vi "Reaction.vi"(5 "Enable potentiostat":bool, 6 "Experiment file path":path, 7 "Potentiostat channel":string(combo)="17158001", 8 "Enable rotation":bool, 9 "Rotation COM":refnum<visa-resource-name>="COM28", 10 "Control parameter":T1={"Pump 1 refill rate (ml/min) "=6.0, "Pump 1 refill volume (mL)"=1.8, "Pump 1 transfer rate (ml/min)"=0.08, "Pump 1 oscill. rate (ml/min)"=0.04, "Vertex potential 1(V)"=-0.5, "Initial potential (V)"=0.0, "Final potential (V)"=0.0, "Cycles"=1, "Delayed time for waiting(s)"=5.0, "Pressure (psi)"=15.0, "Vertex potential 2(V)"=0.0, "Use inital potential?"=TRUE, "Sample name"="", "To waste flow factor"=5.0, "Temperature (C)"=20.0, "Scan rate (V/s)"=10.0, "Use final potential?"=TRUE, "CV current range"="20MA", "Cell to use"="EXTERNAL"} {"Scan rate (V/s)" min=0.0 max=10.0 format="%#_4f"; "Vertex potential 2(V)" min=-5.0 max=5.0 format="%.3f"; "Cycles" min=1 max=30; "Final potential (V)" min=-5.0 format="%_3f"; "Initial potential (V)" min=-5.0 max=5.0 format="%.3f"; "Vertex potential 1(V)" min=-5.0 max=5.0 format="%.3f"; "Pump 1 oscill. rate (ml/min)" format="%#.4f"; "Pump 1 transfer rate (ml/min)" format="%#.4f"; "Pump 1 refill volume (mL)" format="%#.4f"; "Pump 1 refill rate (ml/min)" format="%#.4f"}, 11 "Configured COM ports":T2={"Pump 1 COM"="COM12", "Pump 2 COM"="COM9", "Pump 3 COM"="COM13", "Pump 4 COM"="COM4", "Pump 5 COM"="COM15"}) -> ()   [LabVIEW 2017]
uses:
  C:/Program Files (x86)/Princeton Applied Research/VersaSTAT Development Kit/LabView v2011 Examples/VersaSTATControl.dll
  Program Files (x86)/Princeton Applied Research/VersaSTAT Development Kit/LabView v2011 Examples/VersaSTATControl.dll
  <instrlib>/Harvard Apparatus PHD Ultra Series/Harvard Apparatus PHD Ultra Series.lvlib
  <instrlib>/Princeton potentiostat/Princeton potentiostat.lvlib
panel:
  out "Cell to use":string
  out "CV current range":string
  out "Scan rate (V/s)":dbl
  out "Cycles":i32
  out "Vertex potential 1(V)":dbl
  out "Vertex potential 2(V)":dbl
  out "Initial potential (V)":dbl
  out "Use final potential?":bool
  out "Potentiostat ref.":refnum<k24>
  out "Connect":bool
  out "Temperature (C)":dbl
  out "To waste flow factor":dbl
  out "Sample name":string
  out "Use initial potential?":bool
  out "Pump 5 COM":refnum<visa-resource-name>="COM12"
  out "Final voltage (V)":dbl min=-6.0 max=6.0 format="%.3f"
  out "Pressure (psi)":dbl=15.0
  out "Delayed time for waiting(s)":dbl
  out "Pump 4 COM":refnum<visa-resource-name>="COM12"
  out "Pump 3 COM":refnum<visa-resource-name>="COM12"
  out "Pump 2 COM":refnum<visa-resource-name>="COM12"
  out "Pump 1 COM":refnum<visa-resource-name>="COM12"
  out "Pump 1 oscill. rate (ml/min)":dbl=0.5 format="%#.4f"
  out "Pump 1 transfer rate (ml/min)":dbl=0.15 format="%#.4f"
  out "Pump 1 refill volume (mL)":dbl=1.0 format="%#.4f"
  out "Pump 1 refill rate (ml/min)":dbl=6.0 format="%#.4f"
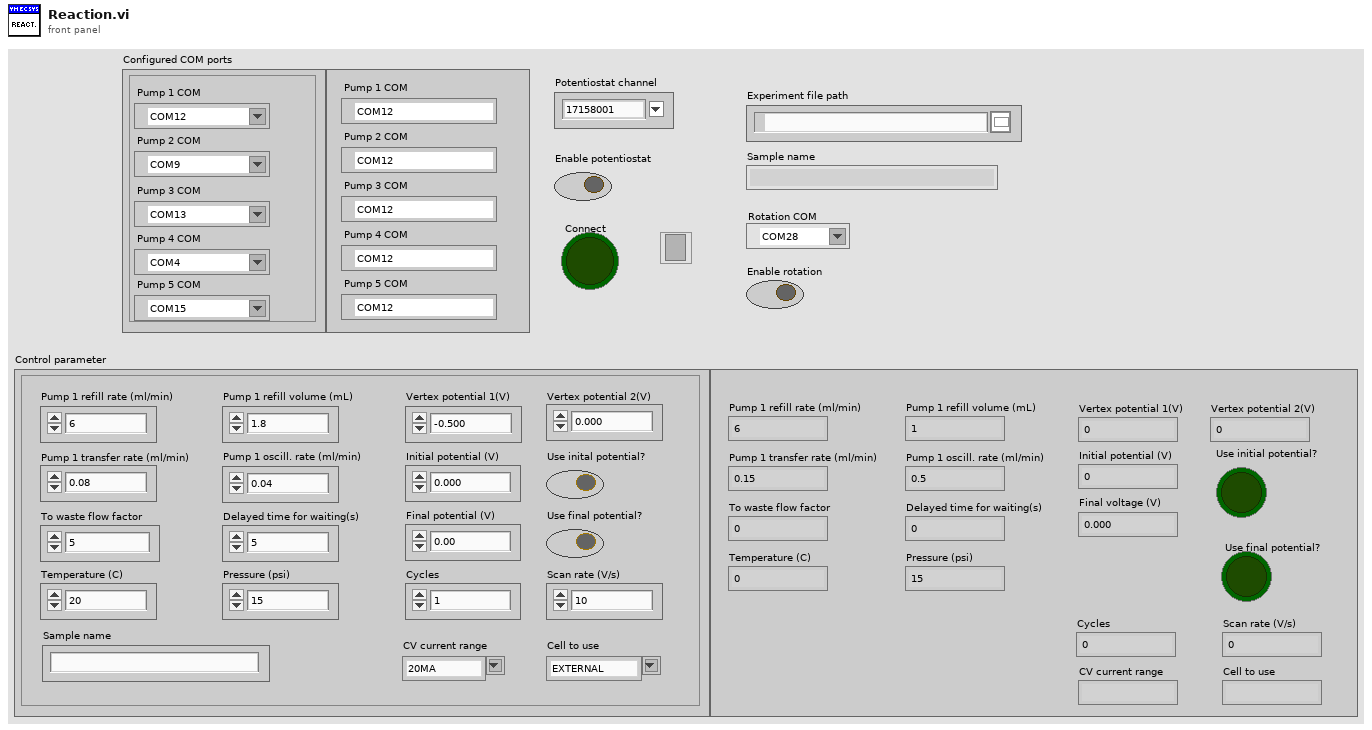
[diagram p1: front panel]
types:
  T1 = cluster{"Pump 1 refill rate (ml/min) ":dbl, "Pump 1 refill volume (mL)":dbl, "Pump 1 transfer rate (ml/min)":dbl, "Pump 1 oscill. rate (ml/min)":dbl, "Vertex potential 1(V)":dbl, "Initial potential (V)":dbl, "Final potential (V)":dbl, "Cycles":i32, "Delayed time for waiting(s)":dbl, "Pressure (psi)":dbl, "Vertex potential 2(V)":dbl, "Use inital potential?":bool, "Sample name":string, "To waste flow factor":dbl, "Temperature (C)":dbl, "Scan rate (V/s)":dbl, "Use final potential?":bool, "CV current range":string, "Cell to use":string}
  T2 = cluster{"Pump 1 COM":refnum<visa-resource-name>, "Pump 2 COM":refnum<visa-resource-name>, "Pump 3 COM":refnum<visa-resource-name>, "Pump 4 COM":refnum<visa-resource-name>, "Pump 5 COM":refnum<visa-resource-name>}
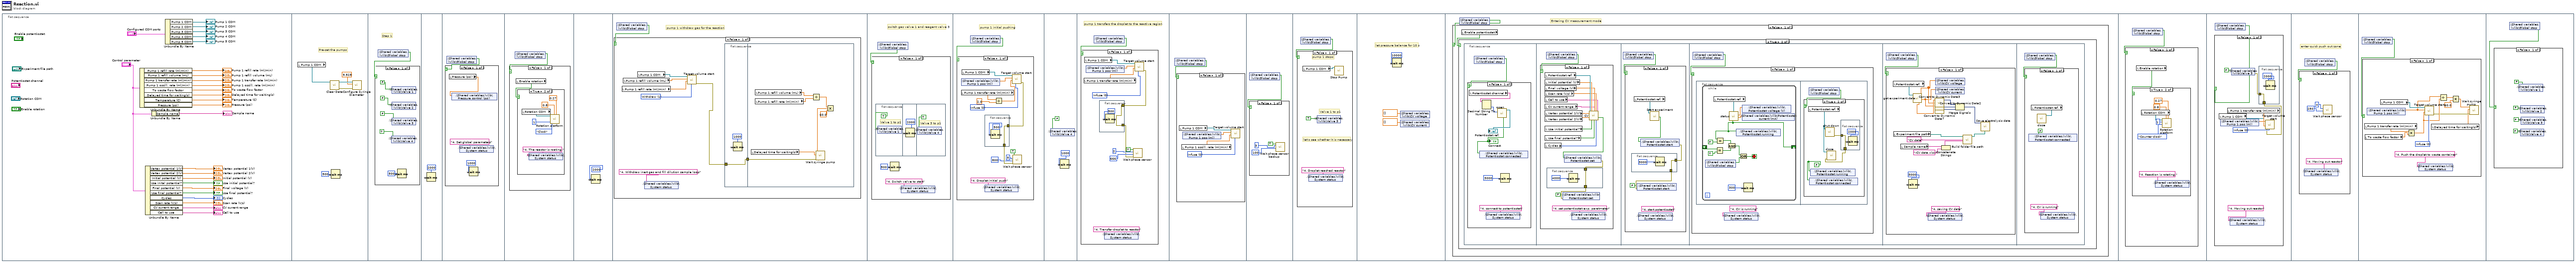
[diagram p0: block diagram]
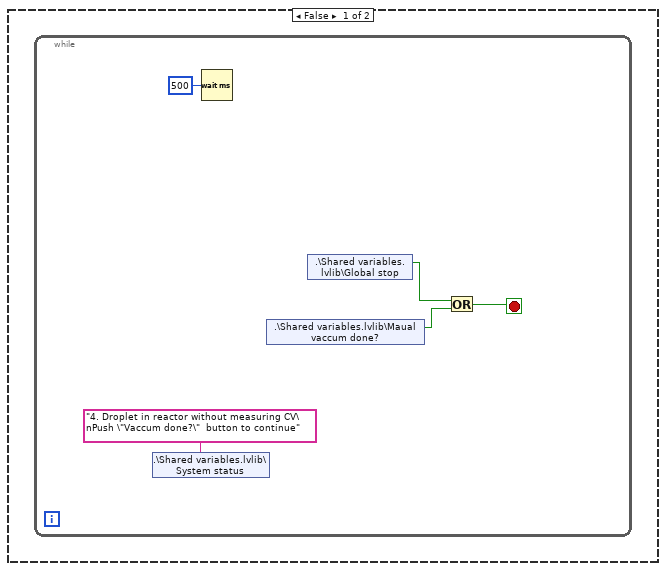
[diagram p13: hidden frame]
diagram:
  n1 = flat-sequence {
    frame #0 {
      n2 = Unbundle By Name("Control parameter") -> ("Pump 1 refill rate (ml/min)"=→"Pump 1 refill rate (ml/min)":dbl, "Pump 1 refill volume (mL)"=→"Pump 1 refill volume (mL)":dbl, "Pump 1 transfer rate (ml/min)"=→"Pump 1 transfer rate (ml/min)":dbl, "Pump 1 oscill. rate (ml/min)"=→"Pump 1 oscill. rate (ml/min)":dbl, "To waste flow factor"=→"To waste flow factor":dbl, "Delayed time for waiting(s)"=→"Delayed time for waiting(s)":dbl, "Temperature (C)"=→"Temperature (C)":dbl, "Pressure (psi)"=→"Pressure (psi)":dbl)
      n3 = Unbundle By Name("Control parameter") -> ("Vertex potential 1(V)"=→"Vertex potential 1(V)":dbl, "Vertex potential 2(V)"=→"Vertex potential 2(V)":dbl, "Initial potential (V)"=→"Initial potential (V)":dbl, "Use inital potential?"=→"Use initial potential?":bool, "Final potential (V)"=→"Final voltage (V)":dbl, "Use final potential?"=→"Use final potential?":bool, "Cycles"=→"Cycles":i32, "Scan rate (V/s)"=→"Scan rate (V/s)":dbl, "CV current range"=→"CV current range":string, "Cell to use"=→"Cell to use":string)
      n4 = Unbundle By Name("Control parameter") -> ("Sample name"=→"Sample name":string)
      n5 = Unbundle By Name("Configured COM ports") -> ("Pump 1 COM"=→"Pump 1 COM":refnum<visa-resource-name>, "Pump 2 COM"=→"Pump 2 COM":refnum<visa-resource-name>, "Pump 3 COM"=→"Pump 3 COM":refnum<visa-resource-name>, "Pump 4 COM"=→"Pump 4 COM":refnum<visa-resource-name>, "Pump 5 COM"=→"Pump 5 COM":refnum<visa-resource-name>)
    }
    frame #1 {
      # "Pre-set the pumps"
      n6 = local read "Pump 1 COM"() -> (w31:refnum<visa-resource-name>)
      n7 = call <instrlib>:"Clear Data.vi"("VISA resource name"=w31) -> ("error out"=w29:errorcluster, "VISA resource name out"=w30:refnum<visa-resource-name>)  [unwired: 9 in]
      n8 = Wait (ms)(milliseconds to wait=u32 500) -> ()  [unwired: 1 out]
      n9 = call <instrlib>:"Configure Syringe Diameter.vi"("error in (no error)"=w29, "Syringe Diameter (20 mm)"=9.525, "VISA resource name"=w30) -> ()  [unwired: 7 in, 2 out]
    }
    frame #2 {
      # "Step 1"
      n10 = shared-variable ".\\Shared variables.lvlib\\Global stop"() -> (w32:bool)  [unwired: 1 in, 1 out]
      n11 = case shown="False" w32 {
        frame False {
          n12 = shared-variable ".\\Shared variables.lvlib\\Valve 4"(TRUE) -> ()  [unwired: 1 in, 1 out]
          n13 = shared-variable ".\\Shared variables.lvlib\\Valve 1"(FALSE) -> ()  [unwired: 1 in, 1 out]
          n14 = shared-variable ".\\Shared variables.lvlib\\Valve 2"(FALSE) -> ()  [unwired: 1 in, 1 out]
          n15 = shared-variable ".\\Shared variables.lvlib\\Valve 3"(FALSE) -> ()  [unwired: 1 in, 1 out]
          n16 = Wait (ms)(milliseconds to wait=u32 500) -> ()  [unwired: 1 out]
        }
        frame True {
        }
      }
    }
    frame #3 {
      n17 = Wait (ms)(milliseconds to wait=u32 2000) -> ()  [unwired: 1 out]
    }
    frame #4 {
      n18 = shared-variable ".\\Shared variables.lvlib\\Global stop"() -> (w39:bool)  [unwired: 1 in, 1 out]
      n19 = case shown="False" w39 {
        frame False {
          n20 = local read "Pressure (psi)"() -> (w42:dbl)
          n21 = shared-variable ".\\Shared variables.lvlib\\Pressure control (psi)"(w42) -> ()  [unwired: 1 in, 1 out]
          n22 = shared-variable ".\\Shared variables.lvlib\\System status"("4. Set global parameters" ("System status")) -> ()  [unwired: 1 in, 1 out]
          n23 = Wait (ms)(milliseconds to wait=u32 1000) -> ()  [unwired: 1 out]
        }
        frame True {
        }
      }
    }
    frame #5 {
      n24 = shared-variable ".\\Shared variables.lvlib\\Global stop"() -> (w43:bool)  [unwired: 1 in, 1 out]
      n25 = case shown="False" w43 {
        frame False {
          n26 = local read "Enable rotation"() -> (w44:bool)
          n27 = case shown="True" w44 {
            frame False {
            }
            frame True {
              n28 = local read "Rotation COM"() -> (w46:refnum<visa-resource-name>)
              n29 = shared-variable ".\\Shared variables.lvlib\\System status"("4. The reactor is roating." ("System status")) -> ()  [unwired: 1 in, 1 out]
              n30 = call "Rotation platform.vi"("Revolution (0-0.5)"=0.27, "Rotation speed (RPM)"=0.8, "Direction"=enum16{"Counter clock", "Clock"}."Clock", "Pump number"=1, "Rotation COM"=w46) -> ()  [unwired: 7 in]
            }
          }
        }
        frame True {
        }
      }
    }
    frame #6 {
      n31 = Wait (ms)(milliseconds to wait=u32 2000) -> ()  [unwired: 1 out]
    }
    frame #7 {
      # "pump 1 withdraw gas for the reaction"
      n32 = shared-variable ".\\Shared variables.lvlib\\Global stop"() -> (w52:bool)  [unwired: 1 in, 1 out]
      n33 = case shown="False" w52 {
        frame False {
          w56 = u16 1 items=["Infuse", "Withdraw"] ("Pump Direction (0:Infuse)")
          n34 = local read "Pump 1 refill rate (ml/min)"() -> (w57:dbl)
          n35 = local read "Pump 1 refill volume (mL)"() -> (w58:dbl)
          n36 = local read "Pump 1 COM"() -> (w55:refnum<visa-resource-name>)
          n37 = shared-variable ".\\Shared variables.lvlib\\System status"("4. Withdraw inert gas and fill dilution sample loop" ("System status")) -> ()  [unwired: 1 in, 1 out]
          n38 = call "Target volume start.vi"("Pump Direction (0:Infuse)"=w56, "Flow Rate (ml/min)"=w57, "Target volume (ml)"=w58, "VISA resource name"=w55) -> ("error out"=w53:errorcluster)  [unwired: 6 in, 1 out]
          n39 = flat-sequence {
            tunnel: [w60] -> w59
            tunnel: w53 -> [w60]
            tunnel: w59 -> [w66]
            frame #0 {
              n40 = Wait (ms)(milliseconds to wait=u32 1000) -> ()  [unwired: 1 out]
            }
            frame #1 {
              n41 = local read "Delayed time for waiting(s)"() -> (w65:dbl)
              n42 = local read "Pump 1 refill volume (mL)"() -> (w68:dbl)
              n43 = local read "Pump 1 refill rate (ml/min)"() -> (w67:dbl)
              n44 = Divide(x=w68, y=w67) -> (x/y=w62:dbl)
              n45 = Multiply(x=w62, y=60.0) -> (x*y=w64:dbl)
              n46 = call "Wait syringe pump.vi"("error in (no error)"=w66, "Delayed time (s)"=w65, "Time Target (s)"=w64) -> ()  [unwired: 8 in, 1 out]
            }
          }
        }
        frame True {
        }
      }
    }
    frame #8 {
      # "switch gas valve 1 and reagent valve 3"
      n47 = shared-variable ".\\Shared variables.lvlib\\Global stop"() -> (w69:bool)  [unwired: 1 in, 1 out]
      n48 = case shown="False" w69 {
        frame False {
          n49 = flat-sequence {
            frame #0 {
              # "Valve 1 to p1"
              n50 = shared-variable ".\\Shared variables.lvlib\\Valve 1"(TRUE) -> ()  [unwired: 1 in, 1 out]
            }
            frame #1 {
              n51 = Wait (ms)(milliseconds to wait=u32 2000) -> ()  [unwired: 1 out]
            }
            frame #2 {
              # "Valve 3 to p1"
              n52 = shared-variable ".\\Shared variables.lvlib\\Valve 4"(TRUE) -> ()  [unwired: 1 in, 1 out]
            }
          }
          n53 = Wait (ms)(milliseconds to wait=u32 500) -> ()  [unwired: 1 out]
          n54 = shared-variable ".\\Shared variables.lvlib\\System status"("4. Switch valve to start" ("System status")) -> ()  [unwired: 1 in, 1 out]
        }
        frame True {
        }
      }
    }
    frame #9 {
      # "pump 1 initial pushing"
      n55 = shared-variable ".\\Shared variables.lvlib\\Global stop"() -> (w75:bool)  [unwired: 1 in, 1 out]
      n56 = case shown="False" w75 {
        frame False {
          w87 = u16 0 items=["Infuse", "Withdraw"] ("Pump Direction (0:Infuse)")
          n57 = shared-variable ".\\Shared variables.lvlib\\Pump 1 pos (ml)"() -> (w78:dbl)  [unwired: 1 in, 1 out]
          n58 = local read "Pump 1 transfer rate (ml/min)"() -> (w83:dbl)
          n59 = local read "Pump 1 COM"() -> (w86:refnum<visa-resource-name>)
          n60 = flat-sequence {
            tunnel: [w88] -> w82
            tunnel: w81 -> [w88]
            frame #0 {
              n61 = Wait (ms)(milliseconds to wait=u32 500) -> ()  [unwired: 1 out]
            }
          }
          n62 = shared-variable ".\\Shared variables.lvlib\\System status"("4. Droplet initial push" ("System status")) -> ()  [unwired: 1 in, 1 out]
          n63 = Divide(x=w83, y=2.0) -> (x/y=w85:dbl)
          n64 = call "Target volume start.vi"("Pump Direction (0:Infuse)"=w87, "Flow Rate (ml/min)"=w85, "Target volume (ml)"=w78, "VISA resource name"=w86) -> ("error out"=w81:errorcluster)  [unwired: 6 in, 1 out]
          n65 = call "Wait phase sensor.vi"("error in (no error)"=w82, "Sensitivity time (ms)"=u32 800 ("milliseconds to wait"), "Phase sensor number"=5, "Sense T/F"=TRUE) -> ()  [unwired: 7 in, 1 out]
        }
        frame True {
        }
      }
    }
    frame #10 {
      n66 = shared-variable ".\\Shared variables.lvlib\\Valve 4"(FALSE) -> ()  [unwired: 1 in, 1 out]
      n67 = Wait (ms)(milliseconds to wait=u32 1000) -> ()  [unwired: 1 out]
    }
    frame #11 {
      # "pump 1 transfers the droplet to the reactive region"
      n68 = shared-variable ".\\Shared variables.lvlib\\Global stop"() -> (w92:bool)  [unwired: 1 in, 1 out]
      n69 = case shown="False" w92 {
        frame False {
          w102 = u16 0 items=["Infuse", "Withdraw"] ("Pump Direction (0:Infuse)")
          n70 = local read "Pump 1 transfer rate (ml/min)"() -> (w100:dbl)
          n71 = local read "Pump 1 COM"() -> (w101:refnum<visa-resource-name>)
          n72 = shared-variable ".\\Shared variables.lvlib\\Pump 1 pos (ml)"() -> (w99:dbl)  [unwired: 1 in, 1 out]
          n73 = flat-sequence {
            tunnel: [w103] -> w93
            tunnel: w98 -> [w103]
            frame #0 {
              n74 = Wait (ms)(milliseconds to wait=u32 500) -> ()  [unwired: 1 out]
            }
          }
          n75 = shared-variable ".\\Shared variables.lvlib\\System status"("4. Transfer droplet to reactor" ("System status")) -> ()  [unwired: 1 in, 1 out]
          n76 = call "Wait phase sensor.vi"("error in (no error)"=w93, "Sensitivity time (ms)"=u32 666 ("milliseconds to wait"), "Phase sensor number"=2, "Sense T/F"=TRUE) -> ()  [unwired: 7 in, 1 out]
          n77 = call "Target volume start.vi"("Pump Direction (0:Infuse)"=w102, "Flow Rate (ml/min)"=w100, "Target volume (ml)"=w99, "VISA resource name"=w101) -> ("error out"=w98:errorcluster)  [unwired: 6 in, 1 out]
        }
        frame True {
        }
      }
    }
    frame #12 {
      n78 = shared-variable ".\\Shared variables.lvlib\\Global stop"() -> (w105:bool)  [unwired: 1 in, 1 out]
      n79 = case shown="False" w105 {
        frame False {
          w106 = u16 0 items=["Infuse", "Withdraw"] ("Pump Direction (0:Infuse)")
          n80 = local read "Pump 1 COM"() -> (w109:refnum<visa-resource-name>)
          n81 = local read "Pump 1 oscill. rate (ml/min)"() -> (w108:dbl)
          n82 = shared-variable ".\\Shared variables.lvlib\\Pump 1 pos (ml)"() -> (w107:dbl)  [unwired: 1 in, 1 out]
          n83 = call "Target volume start.vi"("Pump Direction (0:Infuse)"=w106, "Flow Rate (ml/min)"=w108, "Target volume (ml)"=w107, "VISA resource name"=w109) -> ()  [unwired: 6 in, 2 out]
        }
        frame True {
        }
      }
    }
    frame #13 {
      n84 = shared-variable ".\\Shared variables.lvlib\\Global stop"() -> (w110:bool)  [unwired: 1 in, 1 out]
      n85 = case shown="False" w110 {
        frame False {
          n86 = call "Wait phase sensor backup.vi"("Sensitivity time (ms)"=u32 100 ("milliseconds to wait"), "Phase sensor number"=3, "Sense T/F"=TRUE) -> ()  [unwired: 8 in, 1 out]
        }
        frame True {
        }
      }
    }
    frame #14 {
      n87 = shared-variable ".\\Shared variables.lvlib\\Global stop"() -> (w114:bool)  [unwired: 1 in, 1 out]
      n88 = case shown="False" w114 {
        frame False {
          # "Valve 1 to p1"
          # "let's see whether it is necessary"
          # "pump 1 stops"
          n89 = local read "Pump 1 COM"() -> (w116:refnum<visa-resource-name>)
          n90 = shared-variable ".\\Shared variables.lvlib\\System status"("4. Droplet reached reactor" ("System status")) -> ()  [unwired: 1 in, 1 out]
          n91 = shared-variable ".\\Shared variables.lvlib\\Valve 3"(TRUE) -> ()  [unwired: 1 in, 1 out]
          n92 = call <instrlib>:"Stop Pump.vi"("VISA resource name"=w116) -> ()  [unwired: 9 in, 2 out]
        }
        frame True {
        }
      }
    }
    frame #15 {
      # "let pressure balance for 10 s"
      n93 = Wait (ms)(milliseconds to wait=u32 10000) -> ()  [unwired: 1 out]
      n94 = shared-variable ".\\Shared variables.lvlib\\CV voltage"(dbl[] [] ("CV voltage")) -> ()  [unwired: 1 in, 1 out]
      n95 = shared-variable ".\\Shared variables.lvlib\\CV current"(dbl[] [] ("CV current")) -> ()  [unwired: 1 in, 1 out]
    }
    frame #16 {
      # "Entering CV measurement mode"
      n96 = shared-variable ".\\Shared variables.lvlib\\Global stop"() -> (w121:bool)  [unwired: 1 in, 1 out]
      n97 = case shown="False" w121 {
        frame False {
          n98 = local read "Enable potentiostat"() -> (w122:bool)
          n99 = case shown="True" w122 {
            frame False {
              n100 = while {
                stop <- w123 stop-if-true
                n101 = shared-variable ".\\Shared variables.lvlib\\System status"("4. Droplet in reactor without measuring CV\nPush \"Vaccum done?\"  button to continue" ("System status")) -> ()  [unwired: 1 in, 1 out]
                n102 = Wait (ms)(milliseconds to wait=u32 500) -> ()  [unwired: 1 out]
                n103 = shared-variable ".\\Shared variables.lvlib\\Maual vaccum done?"() -> (w124:bool)  [unwired: 1 in, 1 out]
                n104 = shared-variable ".\\Shared variables.lvlib\\Global stop"() -> (w125:bool)  [unwired: 1 in, 1 out]
                n105 = Or(x=w125, y=w124) -> (x .or. y?=w123:bool)
              }
            }
            frame True {
              n106 = flat-sequence {
                frame #0 {
                  n107 = shared-variable ".\\Shared variables.lvlib\\Global stop"() -> (w128:bool)  [unwired: 1 in, 1 out]
                  n108 = case shown="False" w128 {
                    frame False {
                      n109 = local read "Potentiostat channel"() -> (w131:string)
                      n110 = Decimal String To Number(string=w131) -> (number=w134:i32)  [unwired: 2 in, 1 out]
                      n111 = shared-variable ".\\Shared variables.lvlib\\System status"("4. connect to potentiostat" ("System status")) -> ()  [unwired: 1 in, 1 out]
                      n112 = call <instrlib>:"open.vi"("iSerialNumber"=w134) -> ("Connect"=w132:bool, "reference out"=→"Potentiostat ref.":refnum<k24>)  [unwired: 7 in, 2 out]
                      "Connect" <- w132
                      n113 = shared-variable ".\\Shared variables.lvlib\\Potentiostat connected"(w132) -> ()  [unwired: 1 in, 1 out]
                      n114 = Wait (ms)(milliseconds to wait=u32 3000) -> ()  [unwired: 1 out]
                    }
                    frame True {
                    }
                  }
                }
                frame #1 {
                  n115 = shared-variable ".\\Shared variables.lvlib\\Global stop"() -> (w135:bool)  [unwired: 1 in, 1 out]
                  n116 = case shown="False" w135 {
                    frame False {
                      n117 = local read "Potentiostat ref."() -> (w151:refnum<k24>)
                      n118 = local read "Initial potential (V)"() -> (w148:dbl)
                      n119 = local read "Final voltage (V)"() -> (w147:dbl)
                      n120 = local read "Scan rate (V/s)"() -> (w146:dbl)
                      n121 = local read "Cell to use"() -> (w145:string)
                      n122 = local read "CV current range"() -> (w144:string)
                      n123 = local read "Vertex potential 1(V)"() -> (w143:dbl)
                      n124 = local read "Vertex potential 2(V)"() -> (w142:dbl)
                      n125 = local read "Use initial potential?"() -> (w141:bool)
                      n126 = local read "Use final potential?"() -> (w140:bool)
                      n127 = local read "Cycles"() -> (w139:i32)
                      n128 = flat-sequence {
                        tunnel: [w152] -> w138
                        tunnel: w137 -> [w152]
                        frame #0 {
                          n129 = Wait (ms)(milliseconds to wait=u32 4000) -> ()  [unwired: 1 out]
                        }
                      }
                      n130 = shared-variable ".\\Shared variables.lvlib\\Potentiostat set"(FALSE ("Potentiostat set"), error in=w138) -> ()  [unwired: 1 out]
                      n131 = shared-variable ".\\Shared variables.lvlib\\System status"("4. set potentiostat exp. paratmeter" ("System status")) -> ()  [unwired: 1 in, 1 out]
                      n132 = call <instrlib>:"CV.vi"("reference"=w151, "Vertex potential 1 (V)"=w143, "Vertex potential 2 (V)"=w142, "Initial potential (V)"=w148, "Use initial potential?"=w141, "Final potential (V)"=w147, "Use final potential?"=w140, "Scan rate (V/s)"=w146, "Cycles"=w139, "Cell to use"=w145, "Current range"=w144) -> ("Experiment setup correctly"=w150:bool)  [unwired: 5 in, 3 out]
                      n133 = shared-variable ".\\Shared variables.lvlib\\Potentiostat set"(w150) -> (error out=w137:errorcluster)  [unwired: 1 in]
                    }
                    frame True {
                    }
                  }
                }
                frame #2 {
                  n134 = shared-variable ".\\Shared variables.lvlib\\Global stop"() -> (w154:bool)  [unwired: 1 in, 1 out]
                  n135 = case shown="False" w154 {
                    frame False {
                      n136 = flat-sequence {
                        tunnel: [w161] -> w157
                        tunnel: w156 -> [w161]
                        frame #0 {
                          n137 = Wait (ms)(milliseconds to wait=u32 3000) -> ()  [unwired: 1 out]
                        }
                      }
                      n138 = local read "Potentiostat ref."() -> (w160:refnum<k24>)
                      n139 = shared-variable ".\\Shared variables.lvlib\\Potentiostat start"(FALSE ("Potentiostat start"), error in=w157) -> ()  [unwired: 1 out]
                      n140 = shared-variable ".\\Shared variables.lvlib\\System status"("4. start potentiostat" ("System status")) -> ()  [unwired: 1 in, 1 out]
                      n141 = call <instrlib>:"Start experiment.vi"("reference"=w160) -> ("Start"=w159:bool)  [unwired: 9 in, 1 out]
                      n142 = shared-variable ".\\Shared variables.lvlib\\Potentiostat start"(w159) -> (error out=w156:errorcluster)  [unwired: 1 in]
                    }
                    frame True {
                    }
                  }
                }
                frame #3 {
                  n143 = shared-variable ".\\Shared variables.lvlib\\Global stop"() -> (w163:bool)  [unwired: 1 in, 1 out]
                  n144 = case shown="False" w163 {
                    frame False {
                      n145 = flat-sequence {
                        frame #0 {
                          n146 = while {
                            shift-right: [w176] -> _
                            shift-left: _ -> [w174]
                            stop <- w168 stop-if-true
                            n147 = shared-variable ".\\Shared variables.lvlib\\Global stop"() -> (w169:bool)  [unwired: 1 in, 1 out]
                            n148 = local read "Potentiostat ref."() -> (w177:refnum<k24>)
                            n149 = Equal?(x=w174, y=TRUE) -> (x = y?=w171:bool)
                            n150 = call <instrlib>:"status.vi"("reference"=w177) -> ("Current (A)"=w166:dbl, "Voltage (V)"=w167:dbl, "Experiment running"=w176:bool)  [unwired: 4 in, 4 out]
                            n151 = Equal?(x=w176, y=FALSE) -> (x = y?=w172:bool)
                            n152 = And(x=w172, y=w171) -> (x .and. y?=w170:bool)
                            n153 = shared-variable ".\\Shared variables.lvlib\\Potentiostat running"(w176) -> ()  [unwired: 1 in, 1 out]
                            n154 = Or(x=w170, y=w169) -> (x .or. y?=w168:bool)
                            n155 = shared-variable ".\\Shared variables.lvlib\\Potentiostat voltage (V)"(w167) -> ()  [unwired: 1 in, 1 out]
                            n156 = shared-variable ".\\Shared variables.lvlib\\Potentiostat current (mA)"(w166) -> ()  [unwired: 1 in, 1 out]
                            n157 = Wait (ms)(milliseconds to wait=u32 300) -> ()  [unwired: 1 out]
                          }
                        }
                        frame #1 {
                          n158 = shared-variable ".\\Shared variables.lvlib\\Global stop"() -> (w178:bool)  [unwired: 1 in, 1 out]
                          n159 = case shown="True" w178 {
                            frame False {
                            }
                            frame True {
                              w182 = FALSE ("Potentiostat running")
                              n160 = local read "Potentiostat ref."() -> (w181:refnum<k24>)
                              n161 = shared-variable ".\\Shared variables.lvlib\\Potentiostat connected"(w182) -> ()  [unwired: 1 in, 1 out]
                              n162 = shared-variable ".\\Shared variables.lvlib\\Potentiostat running"(w182) -> ()  [unwired: 1 in, 1 out]
                              n163 = call <instrlib>:"shut down.vi"("reference"=w181) -> ("error out"=w179:errorcluster)  [unwired: 10 in]
                              n164 = call <instrlib>:"close.vi"("error in (no error)"=w180, "reference"=w181) -> ()  [unwired: 9 in, 1 out]
                              n165 = flat-sequence {
                                tunnel: [w183] -> w180
                                tunnel: w179 -> [w183]
                                frame #0 {
                                n166 = Wait (ms)(milliseconds to wait=u32 2000) -> ()  [unwired: 1 out]
                                }
                              }
                            }
                          }
                        }
                      }
                      n167 = shared-variable ".\\Shared variables.lvlib\\System status"("4. CV is running" ("System status")) -> ()  [unwired: 1 in, 1 out]
                    }
                    frame True {
                    }
                  }
                }
                frame #4 {
                  n168 = shared-variable ".\\Shared variables.lvlib\\Global stop"() -> (w185:bool)  [unwired: 1 in, 1 out]
                  n169 = case shown="False" w185 {
                    frame False {
                      n170 = local read "Potentiostat ref."() -> (w201:refnum<k24>)
                      n171 = local read "Experiment file path"() -> (w197:path)
                      n172 = local read "Sample name"() -> (w199:string)
                      n173 = Wait (ms)(milliseconds to wait=u32 3000) -> ()  [unwired: 1 out]
                      n174 = call <instrlib>:"get experiment data.vi"("reference"=w201) -> ("Current (mA)"=w186:dbl[], "Potential (V)"=w187:dbl[], "Time (s)"=w194:dbl[])  [unwired: 6 in, 2 out]
                      n175 = shared-variable ".\\Shared variables.lvlib\\System status"("4. saving CV data" ("System status")) -> ()  [unwired: 1 in, 1 out]
                      n176 = call "Convert to Dynamic Data2"("Array"=w194) -> ("Dynamic Data Type"=w193:dynamicdata)  [unwired: 3 in]
                      n177 = call "Convert to Dynamic Data3"("Array"=w187) -> ("Dynamic Data Type"=w192:dynamicdata)  [unwired: 3 in]
                      n178 = call "Convert to Dynamic Data7"("Array"=w186) -> ("Dynamic Data Type"=w191:dynamicdata)  [unwired: 3 in]
                      n179 = shared-variable ".\\Shared variables.lvlib\\CV voltage"(w187) -> ()  [unwired: 1 in, 1 out]
                      n180 = shared-variable ".\\Shared variables.lvlib\\CV current"(w186) -> ()  [unwired: 1 in, 1 out]
                      n181 = Concatenate Strings(w199, "-CV data.xlsx" ("string")) -> (w200:string)
                      n182 = Merge Signals(w193, w192, w191) -> (w190:dynamicdata)
                      n183 = call "Build folder file path.vi"("File name"=w200, "Folder name"="CV data", "Experiment file path"=w197) -> ("Path"=w198:path)  [unwired: 7 in, 1 out]
                      n184 = call "Save electrolysis data"("Signals"=w190, "Filename"=w198) -> ()  [unwired: 15 in, 3 out]
                    }
                    frame True {
                    }
                  }
                }
                frame #5 {
                  n185 = shared-variable ".\\Shared variables.lvlib\\Global stop"() -> (w202:bool)  [unwired: 1 in, 1 out]
                  n186 = case shown="False" w202 {
                    frame False {
                      n187 = shared-variable ".\\Shared variables.lvlib\\Potentiostat connected"(FALSE ("Potentiostat connected")) -> ()  [unwired: 1 in, 1 out]
                      n188 = local read "Potentiostat ref."() -> (w205:refnum<k24>)
                      n189 = call <instrlib>:"close.vi"("reference"=w205) -> ()  [unwired: 10 in, 1 out]
                      n190 = shared-variable ".\\Shared variables.lvlib\\System status"("4. CV is running" ("System status")) -> ()  [unwired: 1 in, 1 out]
                    }
                    frame True {
                    }
                  }
                }
              }
            }
          }
        }
        frame True {
        }
      }
    }
    frame #17 {
      n191 = shared-variable ".\\Shared variables.lvlib\\Global stop"() -> (w206:bool)  [unwired: 1 in, 1 out]
      n192 = case shown="False" w206 {
        frame False {
          n193 = local read "Enable rotation"() -> (w207:bool)
          n194 = case shown="True" w207 {
            frame False {
            }
            frame True {
              n195 = local read "Rotation COM"() -> (w213:refnum<visa-resource-name>)
              n196 = shared-variable ".\\Shared variables.lvlib\\System status"("4. Reaction is rotating." ("System status")) -> ()  [unwired: 1 in, 1 out]
              n197 = call "Rotation platform.vi"("Revolution (0-0.5)"=0.27, "Rotation speed (RPM)"=0.8, "Direction"=enum16{"Counter clock", "Clock"}."Counter clock", "Pump number"=1, "Rotation COM"=w213) -> ()  [unwired: 7 in]
            }
          }
        }
        frame True {
        }
      }
    }
    frame #18 {
      n198 = shared-variable ".\\Shared variables.lvlib\\Global stop"() -> (w214:bool)  [unwired: 1 in, 1 out]
      n199 = case shown="False" w214 {
        frame False {
          w221 = u16 0 items=["Infuse", "Withdraw"] ("Pump Direction (0:Infuse)")
          n200 = local read "Pump 1 COM"() -> (w219:refnum<visa-resource-name>)
          n201 = shared-variable ".\\Shared variables.lvlib\\Pump 1 pos (ml)"() -> (w222:dbl)  [unwired: 1 in, 1 out]
          n202 = local read "Pump 1 transfer rate (ml/min)"() -> (w220:dbl)
          n203 = shared-variable ".\\Shared variables.lvlib\\System status"("4. Moving out reactor" ("System status")) -> ()  [unwired: 1 in, 1 out]
          n204 = shared-variable ".\\Shared variables.lvlib\\Valve 3"(FALSE ("Valve 1")) -> (error out=w217:errorcluster)  [unwired: 1 in]
          n205 = flat-sequence {
            tunnel: [w223] -> w216
            tunnel: w217 -> [w223]
            frame #0 {
              n206 = Wait (ms)(milliseconds to wait=u32 2000) -> ()  [unwired: 1 out]
            }
          }
          n207 = call "Target volume start.vi"("Pump Direction (0:Infuse)"=w221, "error in (no error)"=w216, "Flow Rate (ml/min)"=w220, "Target volume (ml)"=w222, "VISA resource name"=w219) -> ()  [unwired: 5 in, 2 out]
        }
        frame True {
        }
      }
    }
    frame #19 {
      # "enter quick push out zone"
      n208 = shared-variable ".\\Shared variables.lvlib\\Global stop"() -> (w225:bool)  [unwired: 1 in, 1 out]
      n209 = case shown="False" w225 {
        frame False {
          n210 = shared-variable ".\\Shared variables.lvlib\\System status"("4. Moving out reactor" ("System status")) -> ()  [unwired: 1 in, 1 out]
          n211 = call "Wait phase sensor.vi"("Sensitivity time (ms)"=u32 250 ("milliseconds to wait"), "Phase sensor number"=4) -> ()  [unwired: 9 in, 1 out]
        }
        frame True {
        }
      }
    }
    frame #20 {
      n212 = shared-variable ".\\Shared variables.lvlib\\Global stop"() -> (w229:bool)  [unwired: 1 in, 1 out]
      n213 = case shown="False" w229 {
        frame False {
          w240 = u16 0 items=["Infuse", "Withdraw"] ("Pump Direction (0:Infuse)")
          n214 = local read "Pump 1 transfer rate (ml/min)"() -> (w239:dbl)
          n215 = local read "To waste flow factor"() -> (w230:dbl)
          n216 = shared-variable ".\\Shared variables.lvlib\\Pump 1 pos (ml)"() -> (w237:dbl)  [unwired: 1 in, 1 out]
          n217 = local read "Pump 1 COM"() -> (w241:refnum<visa-resource-name>)
          n218 = Multiply(x=w239, y=w230) -> (x*y=w236:dbl)
          n219 = shared-variable ".\\Shared variables.lvlib\\System status"("4. Push the droplet to waste container" ("System status")) -> ()  [unwired: 1 in, 1 out]
          n220 = call "Target volume start.vi"("Pump Direction (0:Infuse)"=w240, "Flow Rate (ml/min)"=w236, "Target volume (ml)"=w237, "VISA resource name"=w241) -> ("error out"=w233:errorcluster)  [unwired: 6 in, 1 out]
          n221 = local read "Delayed time for waiting(s)"() -> (w232:dbl)
          n222 = Divide(x=w237, y=w236) -> (x/y=w238:dbl)
          n223 = Multiply(x=w238, y=60.0) -> (x*y=w234:dbl)
          n224 = call "Wait syringe pump.vi"("error in (no error)"=w233, "Delayed time (s)"=w232, "Time Target (s)"=w234) -> ()  [unwired: 8 in, 1 out]
        }
        frame True {
        }
      }
    }
    frame #21 {
      n225 = shared-variable ".\\Shared variables.lvlib\\Global stop"() -> (w242:bool)  [unwired: 1 in, 1 out]
      n226 = case shown="False" w242 {
        frame False {
          n227 = shared-variable ".\\Shared variables.lvlib\\Valve 1"(FALSE ("Valve 1")) -> ()  [unwired: 1 in, 1 out]
          n228 = shared-variable ".\\Shared variables.lvlib\\Valve 4"(FALSE ("Valve 3")) -> ()  [unwired: 1 in, 1 out]
          n229 = shared-variable ".\\Shared variables.lvlib\\Valve 2"(FALSE ("Valve 2")) -> ()  [unwired: 1 in, 1 out]
          n230 = shared-variable ".\\Shared variables.lvlib\\Valve 3"(FALSE ("Valve 3")) -> ()  [unwired: 1 in, 1 out]
        }
        frame True {
        }
      }
    }
  }
